vi "Configure Ramp Time Query.vi"(7 "Mode":T2 items=["AC", "DC", "IR"], 8 "error in (no error)":errorcluster, 10 "Step":T1=1 min=1 max=99 step=1, 11 "VISA resource name":refnum<visa-resource-name>) -> (0 "error out":errorcluster, 2 "Ramp Time value [s]":string, 3 "VISA resource name out":refnum<visa-resource-name>)   [LabVIEW 2025]
uses:
  <instrlib>/Chrome 19025/Public/Utility/Type Def/steps--numeric.ctl
  <instrlib>/Chrome 19025/Public/Utility/Type Def/AC-DC-IR modes--ring.ctl
panel:
  # "Ramp Time query"
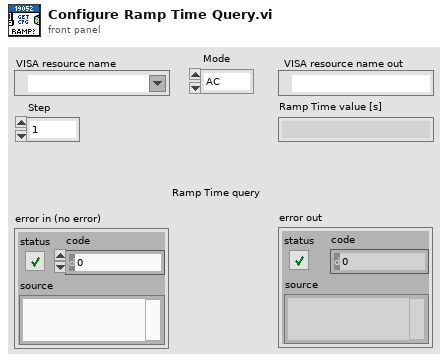
[diagram p1: front panel]
types:
  T1 = typedef "Chrome 19025.lvlib/steps--numeric.ctl" = u8
  T2 = typedef "Chrome 19025.lvlib/AC-DC-IR modes--ring.ctl" = u16
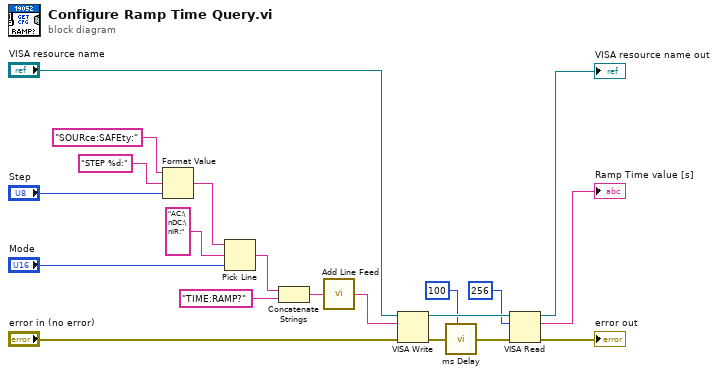
[diagram p0: block diagram]
diagram:
  n1 = Format Value(string ("")="SOURce:SAFEty:", format string="STEP %d:", value (0)="Step") -> (output string=w14:string)
  n2 = Pick Line(string ("")=w14, multi-line string="AC:\nDC:\nIR:", line index="Mode") -> (output string=w11:string)
  n3 = Concatenate Strings(w11, "TIME:RAMP?" ("format string")) -> (w13:string)
  n4 = call <instrlib>:"Add Line Feed.vi"("Command string"=w13) -> ("Concatenated string"=w8:string)  [unwired: 4 in]
  n5 = VISA Write(VISA resource name="VISA resource name", write buffer=w8, error in (no error)="error in (no error)") -> (VISA resource name out=w20:refnum<visa-resource-name>, error out=w3:errorcluster)  [unwired: 1 out]
  n6 = call <instrlib>:"ms Delay.vi"("miliseconds to wait"=u32 100 ("Time Delay ms"), "error in (no error)"=w3) -> ("error out"=w2:errorcluster)  [unwired: 6 in, 1 out]
  n7 = VISA Read(VISA resource name=w20, byte count=u32 256, error in (no error)=w2) -> (VISA resource name out=→"VISA resource name out":refnum<visa-resource-name>, read buffer=→"Ramp Time value [s]":string, error out=→"error out":errorcluster)  [unwired: 1 out]
